vi "S2P GENERATE.vi"() -> ()   [LabVIEW 2011]
uses:
  database/Fields/Field Record.ctl
  database/Fields/Field DataTypes.ctl
  database/Fields/Field NextItem.ctl
panel:
  out "DESTINATION DIRECTORY":path caption="selected path"
  in  "System or ALL Combined Fields":T1[](array[typedef])=[{"ixField"=178, "iSequenceOrder"=0, "sxFieldId"="Test_Station", "sxSequenceId"="", "sDisplayName"="Test Station", "sValue"="", "sUnits"="", "nDataType"=enum."text", "nNextItem"=enum."Reset", "fSystem"=TRUE, "fSystemValue"=TRUE, "fRequired"=TRUE, "fSetAtTest"=TRUE, "fTestField"=FALSE, "fDeleted"=FALSE, "fIndexed"=TRUE, "fFreeList"=FALSE}, {"ixField"=169, "iSequenceOrder"=0, "sxFieldId"="Model_Number", "sxSequenceId"="", "sDisplayName"="Model Number", "sValue"="", "sUnits"="", "nDataType"=enum."text", "nNextItem"=enum."Reset", "fSystem"=TRUE, "fSystemValue"=FALSE, "fRequired"=TRUE, "fSetAtTest"=TRUE, "fTestField"=FALSE, "fDeleted"=FALSE, "fIndexed"=TRUE, "fFreeList"=FALSE}, {"ixField"=170, "iSequenceOrder"=0, "sxFieldId"="Test_Run", "sxSequenceId"="", "sDisplayName"="Test Run", "sValue"="", "sUnits"="", "nDataType"=enum."numeric", "nNextItem"=enum."Reset", "fSystem"=TRUE, "fSystemValue"=TRUE, "fRequired"=TRUE, "fSetAtTest"=TRUE, "fTestField"=FALSE, "fDeleted"=FALSE, "fIndexed"=TRUE, "fFreeList"=FALSE}, {"ixField"=171, "iSequenceOrder"=0, "sxFieldId"="Start_Timestamp", "sxSequenceId"="", "sDisplayName"="Start Timestamp", "sValue"="", "sUnits"="", "nDataType"=enum."timestamp", "nNextItem"=enum."Reset", "fSystem"=TRUE, "fSystemValue"=TRUE, "fRequired"=TRUE, "fSetAtTest"=TRUE, "fTestField"=FALSE, "fDeleted"=FALSE, "fIndexed"=TRUE, "fFreeList"=FALSE}, {"ixField"=172, "iSequenceOrder"=0, "sxFieldId"="End_Timestamp", "sxSequenceId"="", "sDisplayName"="End Timestamp", "sValue"="", "sUnits"="", "nDataType"=enum."timestamp", "nNextItem"=enum."Reset", "fSystem"=TRUE, "fSystemValue"=TRUE, "fRequired"=TRUE, "fSetAtTest"=TRUE, "fTestField"=FALSE, "fDeleted"=FALSE, "fIndexed"=TRUE, "fFreeList"=FALSE}, {"ixField"=173, "iSequenceOrder"=0, "sxFieldId"="Test_Status", "sxSequenceId"="", "sDisplayName"="Test Status", "sValue"="Done\tFail\tPass\tAbort\tError\tDone\tPass by Sample\tFail by Sample\tPass Override\tFail Override\tNot Tested", "sUnits"="", "nDataType"=enum."list", "nNextItem"=enum."Reset", "fSystem"=TRUE, "fSystemValue"=TRUE, "fRequired"=TRUE, "fSetAtTest"=TRUE, "fTestField"=FALSE, "fDeleted"=FALSE, "fIndexed"=TRUE, "fFreeList"=FALSE}, {"ixField"=174, "iSequenceOrder"=0, "sxFieldId"="Test_Type", "sxSequenceId"="", "sDisplayName"="Test Type", "sValue"="", "sUnits"="", "nDataType"=enum."text", "nNextItem"=enum."Reset", "fSystem"=TRUE, "fSystemValue"=TRUE, "fRequired"=TRUE, "fSetAtTest"=TRUE, "fTestField"=FALSE, "fDeleted"=FALSE, "fIndexed"=TRUE, "fFreeList"=FALSE}, {"ixField"=168, "iSequenceOrder"=0, "sxFieldId"="Serial_Number", "sxSequenceId"="", "sDisplayName"="Serial Number", "sValue"="", "sUnits"="", "nDataType"=enum."text", "nNextItem"=enum."Reset", "fSystem"=TRUE, "fSystemValue"=FALSE, "fRequired"=TRUE, "fSetAtTest"=TRUE, "fTestField"=FALSE, "fDeleted"=FALSE, "fIndexed"=TRUE, "fFreeList"=FALSE}, {"ixField"=176, "iSequenceOrder"=0, "sxFieldId"="Operator", "sxSequenceId"="", "sDisplayName"="Operator", "sValue"="", "sUnits"="", "nDataType"=enum."text", "nNextItem"=enum."Reset", "fSystem"=TRUE, "fSystemValue"=TRUE, "fRequired"=TRUE, "fSetAtTest"=TRUE, "fTestField"=FALSE, "fDeleted"=FALSE, "fIndexed"=TRUE, "fFreeList"=FALSE}, {"ixField"=3498, "iSequenceOrder"=0, "sxFieldId"="Spartan_Version_Current", "sxSequenceId"="", "sDisplayName"="Spartan Version Current", "sValue"="", "sUnits"="", "nDataType"=enum."text", "nNextItem"=enum."Reset", "fSystem"=TRUE, "fSystemValue"=TRUE, "fRequired"=TRUE, "fSetAtTest"=TRUE, "fTestField"=FALSE, "fDeleted"=FALSE, "fIndexed"=TRUE, "fFreeList"=FALSE}, {"ixField"=179, "iSequenceOrder"=0, "sxFieldId"="Company", "sxSequenceId"="", "sDisplayName"="Company", "sValue"="Summitek Instruments", "sUnits"="", "nDataType"=enum."text", "nNextItem"=enum."Reset", "fSystem"=TRUE, "fSystemValue"=FALSE, "fRequired"=TRUE, "fSetAtTest"=FALSE, "fTestField"=FALSE, "fDeleted"=FALSE, "fIndexed"=TRUE, "fFreeList"=FALSE}, {"ixField"=232, "iSequenceOrder"=0, "sxFieldId"="Step_Number", "sxSequenceId"="", "sDisplayName"="Step Number", "sValue"="", "sUnits"="", "nDataType"=enum."numeric", "nNextItem"=enum."Reset", "fSystem"=TRUE, "fSystemValue"=TRUE, "fRequired"=TRUE, "fSetAtTest"=TRUE, "fTestField"=FALSE, "fDeleted"=FALSE, "fIndexed"=TRUE, "fFreeList"=FALSE}, {"ixField"=233, "iSequenceOrder"=0, "sxFieldId"="Step_Tag", "sxSequenceId"="", "sDisplayName"="Step Tag", "sValue"="", "sUnits"="", "nDataType"=enum."text", "nNextItem"=enum."Reset", "fSystem"=TRUE, "fSystemValue"=TRUE, "fRequired"=TRUE, "fSetAtTest"=TRUE, "fTestField"=FALSE, "fDeleted"=FALSE, "fIndexed"=TRUE, "fFreeList"=FALSE}, {"ixField"=529, "iSequenceOrder"=0, "sxFieldId"="Test_Version", "sxSequenceId"="", "sDisplayName"="Test Version", "sValue"="", "sUnits"="", "nDataType"=enum."text", "nNextItem"=enum."Reset", "fSystem"=TRUE, "fSystemValue"=TRUE, "fRequired"=TRUE, "fSetAtTest"=TRUE, "fTestField"=FALSE, "fDeleted"=FALSE, "fIndexed"=TRUE, "fFreeList"=FALSE}, {"ixField"=593, "iSequenceOrder"=0, "sxFieldId"="Test_Station_Name", "sxSequenceId"="", "sDisplayName"="Test Station Name", "sValue"="", "sUnits"="", "nDataType"=enum."text", "nNextItem"=enum."Reset", "fSystem"=TRUE, "fSystemValue"=TRUE, "fRequired"=TRUE, "fSetAtTest"=TRUE, "fTestField"=FALSE, "fDeleted"=FALSE, "fIndexed"=TRUE, "fFreeList"=FALSE}, {"ixField"=3452, "iSequenceOrder"=0, "sxFieldId"="Spartan_Version_Created", "sxSequenceId"="", "sDisplayName"="Spartan Version Created", "sValue"="", "sUnits"="", "nDataType"=enum."text", "nNextItem"=enum."Reset", "fSystem"=TRUE, "fSystemValue"=TRUE, "fRequired"=TRUE, "fSetAtTest"=TRUE, "fTestField"=FALSE, "fDeleted"=FALSE, "fIndexed"=TRUE, "fFreeList"=FALSE}, {"ixField"=175, "iSequenceOrder"=0, "sxFieldId"="Test_Sequence", "sxSequenceId"="", "sDisplayName"="Test Sequence", "sValue"="", "sUnits"="", "nDataType"=enum."text", "nNextItem"=enum."Reset", "fSystem"=TRUE, "fSystemValue"=TRUE, "fRequired"=TRUE, "fSetAtTest"=TRUE, "fTestField"=FALSE, "fDeleted"=FALSE, "fIndexed"=TRUE, "fFreeList"=FALSE}]
  out "error out":errorcluster
  # "Instructions: \nYou will be prompted to select the data files to create the S2P files from.\nYou can select several files at once using the control or shift keys. \n\nNext, You will prompted for the destination directory for the S2P files. \n\nAll test runs for each file will be created."
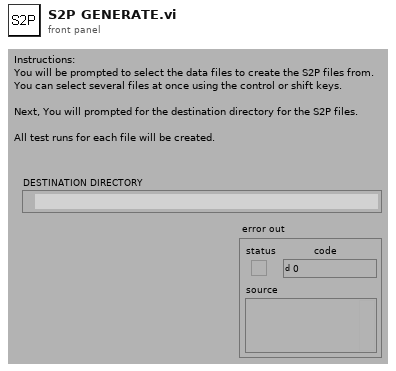
[diagram p1: front panel]
types:
  T1 = typedef "Field Record.ctl" = cluster{"ixField":i32, "iSequenceOrder":i32, "sxFieldId":string, "sxSequenceId":string, "sDisplayName":string, "sValue":string, "sUnits":string, "nDataType":T2, "nNextItem":T3, "fSystem":bool, "fSystemValue":bool, "fRequired":bool, "fSetAtTest":bool, "fTestField":bool, "fDeleted":bool, "fIndexed":bool, "fFreeList":bool}
  T2 = typedef "Field DataTypes.ctl" = enum32{"text", "numeric", "list", "timestamp", "boolean"}
  T3 = typedef "Field NextItem.ctl" = enum32{"Reset", "Retain", "Auto-Increment"}
  T4 = typedef "TDMS File.ctl" = cluster{"File Path":path, "Run Data":T5[], "Serial Number":string, "Model Number":string, "Test Type":string}
  T5 = typedef "TDMS Run.ctl" = cluster{"Channel Data":T6[], "Custom Fields":T1[], "Run ID":string}
  T6 = typedef "TDMS Channel (Sxx).ctl" = cluster{"Channel Name":string, "Waveform":dbl[], "Unit":string, "List value":string}
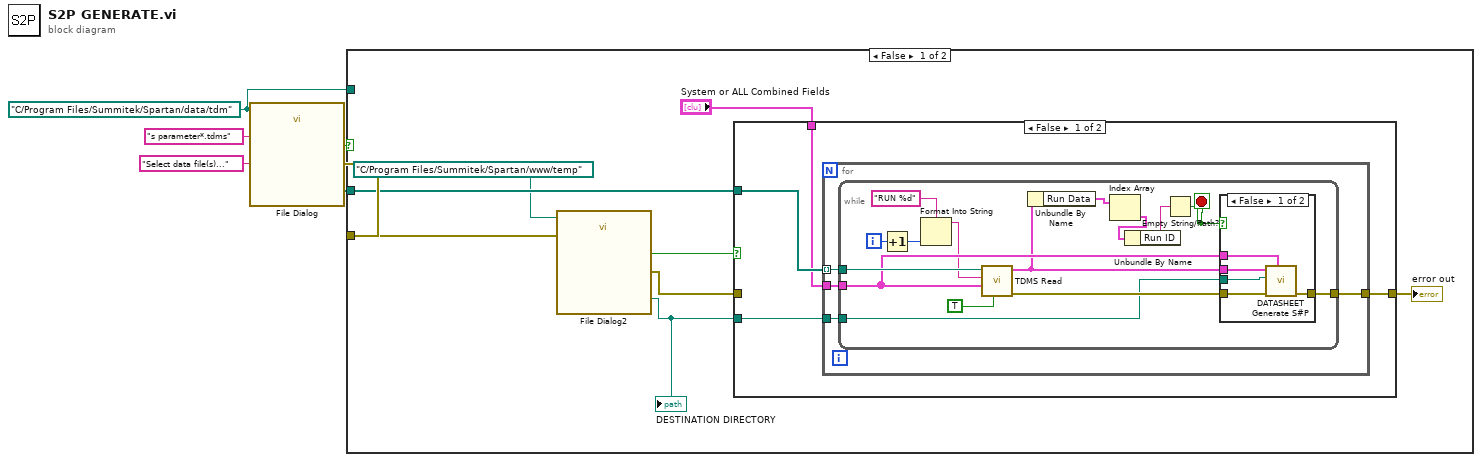
[diagram p0: block diagram]
diagram:
  w2 = path "C:/Program Files/Summitek/Spartan/data/tdm" ("start path")
  n1 = call "File Dialog"("start path"=w2, "prompt"="Select data file(s)...", "pattern (all files)"="s parameter*.tdms") -> ("selected paths"=w3:path[], "cancelled"=w4:bool, "error out"=w1:errorcluster)  [unwired: 9 in, 1 out]
  n2 = case shown="False" w4 {
    tunnel: w3 -> [w14 _]
    tunnel: w2 -> [_ _]
    tunnel: w1 -> [w8 _]
    frame False {
      n3 = call "File Dialog2"("start path"=path "C:/Program Files/Summitek/Spartan/www/temp", "error in"=w8) -> ("selected path"=w11:path, "cancelled"=w10:bool, "error out"=w9:errorcluster)  [unwired: 10 in, 1 out]
      "DESTINATION DIRECTORY" <- w11
      n4 = case shown="False" w10 {
        tunnel: w14 -> [w18 _]
        tunnel: "System or ALL Combined Fields" -> [w17 _]
        tunnel: [w16 w44] -> w12
        tunnel: w11 -> [w15 _]
        tunnel: w9 -> [_ w44]
        frame False {
          n5 = for {
            tunnel: w18 -> [w22] mode=indexing
            tunnel: w17 -> [w21]
            tunnel: [w20] -> w16
            tunnel: w15 -> [w19]
            n6 = while {
              tunnel: w22 -> [w35]
              tunnel: w21 -> [w34]
              tunnel: [w33] -> w20
              tunnel: w19 -> [w23]
              i -> [w30]
              stop <- w24 stop-if-true
              n7 = Increment(x=w30) -> (x+1=w28:i32)
              n8 = Format Into String(format string="RUN %d" ("Run String"), w28) -> (resulting string=w29:string)  [unwired: 2 in, 1 out]
              n9 = call "TDMS Read.vi"("Load Fields?"=TRUE, "System or ALL Combined Fields"=w34, "Run String"=w29, "TDM File Path"=w35) -> ("error out"=w36:errorcluster, "File Information"=w32:T4)  [unwired: 4 in, 2 out]
              n10 = Unbundle By Name(w32) -> ("Run Data"=w27:T5[])
              n11 = Index Array(array=w27) -> (element=w26:T5)  [unwired: 1 in]
              n12 = Unbundle By Name(w26) -> ("Run ID"=w25:string)
              n13 = Empty String/Path?(string/path=w25) -> (empty?=w24:bool)
              n14 = case shown="False" w24 {
                tunnel: w36 -> [w42 w43]
                tunnel: w34 -> [w41 _]
                tunnel: [w40 w43] -> w33
                tunnel: w32 -> [w39 _]
                tunnel: w23 -> [w38 _]
                frame False {
                  n15 = call "DATASHEET Generate S#P.vi"("System or ALL Combined Fields"=w41, "error in (no error)"=w42, "Destination Directory (Temp)"=w38, "File Information"=w39) -> ("error out"=w40:errorcluster)  [unwired: 6 in, 1 out]
                }
                frame True {
                }
              }
            }
          }
        }
        frame True {
        }
      }
      "error out" <- w12
    }
    frame True {
    }
  }
